vi "Send M1M3 Detail State Event.vi"(8 "error in (no error)":errorcluster, 10 "logevent_DetailedState":T1, 11 "M1M3 Support Events in":refnum<class "M1M3 Support Events.lvclass">) -> (0 "error out":errorcluster, 3 "M1M3 Support Events out":refnum<class "M1M3 Support Events.lvclass">)   [LabVIEW 2016, in "M1M3 Support Events.lvclass"]
uses:
  M1M3 Support Events.lvclass
  SALLV_m1m3/DataTypes/logevent_DetailedState.ctl
  M1M3 Support Events.lvclass/M1M3 Support Events.ctl
  SALLV_m1m3/SALLV_m1m3.lvlib
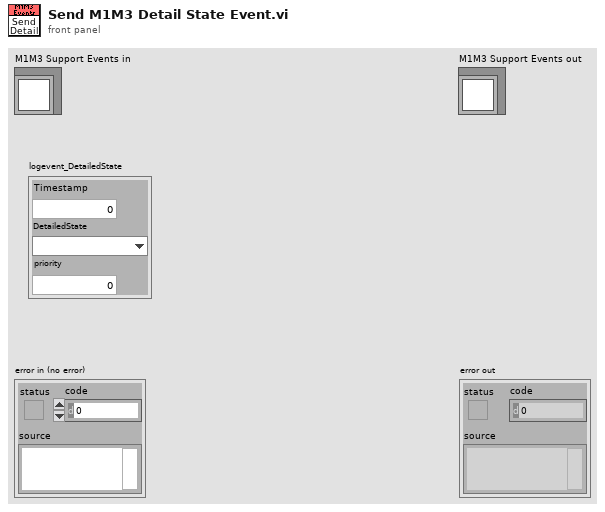
[diagram p1: front panel]
types:
  T1 = typedef "SALLV_m1m3.lvlib/logevent_DetailedState.ctl" = cluster{"Timestamp":dbl, "DetailedState":enum16{"", "DetailedState_DetailedStates_DisabledState", "DetailedState_DetailedStates_EnabledState", "DetailedState_DetailedStates_FaultState", "DetailedState_DetailedStates_OfflineState", "DetailedState_DetailedStates_StandbyState", "DetailedState_DetailedStates_ParkedState", "DetailedState_DetailedStates_RaisingState", "DetailedState_DetailedStates_ActiveState", "DetailedState_DetailedStates_LoweringState", "DetailedState_DetailedStates_EngineeringState", "DetailedState_DetailedStates_ParkedEngineeringState", "DetailedState_DetailedStates_RaisingEngineeringState", "DetailedState_DetailedStates_ActiveEngineeringState", "DetailedState_DetailedStates_LoweringEngineeringState", "DetailedState_DetailedStates_LoweringFaultState", "DetailedState_DetailedStates_ProfileHardpointCorrectionState"}, "priority":i32}
  T2 = typedef "M1M3SupportEUI_TypeDefs.lvlib/M1M3 Support Events.ctl" = cluster{"Inclinometer  Data":refnum<user-event>, "IMS Data":refnum<user-event>, "SAL Connected":refnum<user-event>, "Accelerometer Data":refnum<user-event>, "OuterLoop Data":refnum<user-event>, "ErrorCode Event":refnum<user-event>, "InterlockStatus Event":refnum<user-event>, "InterlockWarning Event":refnum<user-event>, "Gyro Data":refnum<user-event>, "HP Actuator Info Event":refnum<user-event>, " FA Info Event":refnum<user-event>, "HP Monitor Info Event":refnum<user-event>, "FA Data":refnum<user-event>, "HP Actuator data":refnum<user-event>, "HP Monitor data":refnum<user-event>, "Air Supply Status Event":refnum<user-event>, "Air Supply Warning Event":refnum<user-event>, "Power Data":refnum<user-event>, "PID Data":refnum<user-event>, "PID Info Event":refnum<user-event>, "Power Status Event":refnum<user-event>, "Power Supply Status Event":refnum<user-event>, "Power Warning Event":refnum<user-event>, "Summary State Event":refnum<user-event>, "Detailed State Event":refnum<user-event>, "FA Force Warning Event":refnum<user-event>, "FA Warning Event":refnum<user-event>, "FA State Event":refnum<user-event>, "Applied AberrationForces Event":refnum<user-event>, "Applied Acceleration Forcces Event":refnum<user-event>, "Applied Azimuth Forces Event":refnum<user-event>, "Applied Active Optic Forces Event":refnum<user-event>, "Applied Balance Forces Event":refnum<user-event>, "Applied Cylinder Forces Event":refnum<user-event>, "Applied Elevation Forces Event":refnum<user-event>, "Applied Forces Event":refnum<user-event>, "Applied Offset Forces Event":refnum<user-event>, "Applied Static Forces Event":refnum<user-event>, "Applied Thermal Forces Event":refnum<user-event>, "Applied Velocity Forces Event":refnum<user-event>, "Rejected Aberration Force Event":refnum<user-event>, "Rejected Acceleration Forces Event":refnum<user-event>, "Rejected Active Optic Forces Event":refnum<user-event>, "Rejected Azimuth Forces Event":refnum<user-event>, "Rejected Balance Forces Event":refnum<user-event>, "Rejected Cylinder Forces Event":refnum<user-event>, "Rejected Elevation Forces Event":refnum<user-event>, "Rejected Forces Event":refnum<user-event>, "Rejected Offset Forces Event":refnum<user-event>, "Rejected Static Forces Event":refnum<user-event>, "Rejected Thermal Forces Event":refnum<user-event>, "Rejected Velocity Forces Event":refnum<user-event>, "Command Rejection Event":refnum<user-event>, "Setting Verions Event":refnum<user-event>, "Settings Applied Event":refnum<user-event>, "HP Actuator State Event":refnum<user-event>, "HP Actuator Warning Event":refnum<user-event>, "HP Monitor State Event":refnum<user-event>, "HP Monitor Warning Event":refnum<user-event>, "Accelerometer Warning Event":refnum<user-event>, "Applied Settings Match Start Event":refnum<user-event>, "Cell Light Status Event ":refnum<user-event>, "Cell Light Warning Event":refnum<user-event>, "Displacement Sensor Warning Event":refnum<user-event>, "Force Setpoint Warning Event":refnum<user-event>, "Gyro Warning Event ":refnum<user-event>, "ILC Warning Event ":refnum<user-event>, "Inclinometer Sensor Warning Event ":refnum<user-event>}
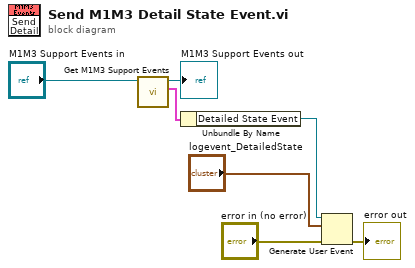
[diagram p0: block diagram]
diagram:
  n1 = call "Get M1M3 Support Events.vi"("M1M3 Support Events in"="M1M3 Support Events in") -> ("M1M3 Support Events"=w7:T2, "M1M3 Support Events out"=→"M1M3 Support Events out":refnum<class "M1M3 Support Events.lvclass">)  [unwired: 9 in]
  n2 = Unbundle By Name(w7) -> ("Detailed State Event"=w2:refnum<user-event>)
  n3 = Generate User Event(user event=w2, event data cluster="logevent_DetailedState", error in="error in (no error)") -> (error out=→"error out":errorcluster)  [unwired: 1 in, 1 out]
